vi "setGlobleVariablesFromJoysticks.vi"(10 "Buttons":bool[](array[boolean]), 11 "Buttons 2":bool[](array[boolean])) -> ()   [LabVIEW 2014]
uses:
  LabVIEW Data/2015 Beta Robot Project/Robot Global Data.vi
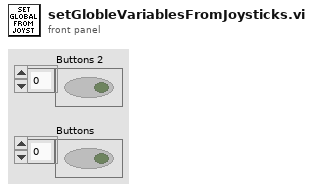
[diagram p1: front panel]
types:
  T1 = cluster{"[0]":bool, "[1]":bool, "[2]":bool, "[3]":bool, "[4]":bool, "[5]":bool, "[6]":bool, "[7]":bool, "[8]":bool}
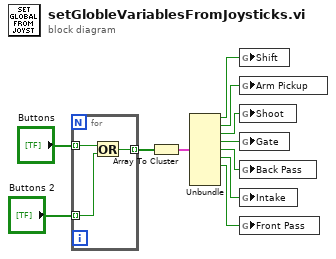
[diagram p0: block diagram]
diagram:
  n1 = for {
    tunnel: "Buttons" -> [w14] mode=indexing
    tunnel: "Buttons 2" -> [w13] mode=indexing
    tunnel: [w12] -> w10 mode=indexing
    n2 = Or(x=w14, y=w13) -> (x .or. y?=w12:bool)
  }
  n3 = Array To Cluster(array=w10) -> (cluster=w7:T1)
  n4 = Unbundle(w7) -> ("[0]"=w8:bool, "[1]"=w6:bool, "[2]"=w5:bool, "[3]"=w4:bool, "[4]"=w3:bool, "[5]"=w2:bool, "[6]"=w1:bool)  [unwired: 2 out]
  n5 = global write "Robot Global Data.vi" "Shift"(w8) -> ()
  n6 = global write "Robot Global Data.vi" "Arm Pickup"(w6) -> ()
  n7 = global write "Robot Global Data.vi" "Shoot"(w5) -> ()
  n8 = global write "Robot Global Data.vi" "Gate"(w4) -> ()
  n9 = global write "Robot Global Data.vi" "Back Pass"(w3) -> ()
  n10 = global write "Robot Global Data.vi" "Intake"(w2) -> ()
  n11 = global write "Robot Global Data.vi" "Front Pass"(w1) -> ()
